vi "ENCODERS AUTO SUBVI.vi"   [LabVIEW 2011]
uses:
  Robot Global Data.vi
types:
  T1 = typedef "WPI_RobotDriveDevRef.ctl" = cluster{"DevStatus":errorcluster, "Motors[]":T2[], "Square Inputs":bool, "Max Output":dbl, "Isochronous":bool}
  T2 = typedef "WPI_MotorControlDeviceRef.ctl" = cluster{"DeviceStatus":errorcluster, "Type":enum16{"PWM", "CAN"}, "PWM":cluster{"Digital Module":T3, "PWM Channel":T4, "DeadBand":T5}, "CAN":cluster{"Device Number":u8, "Control Mode":T6, "Semaphore":T7, "Max Vout":dbl}, "Invert":bool, "TransformRef":T8, "InvTransformRef":T8}
  T3 = typedef "FPGA_TypedefDigitalModule.ctl" = enum16{"Digital Module 1", "Digital Module 2"}
  T4 = typedef "FPGA_DIOPWMChannel.ctl" = enum8{"PWM 1", "PWM 2", "PWM 3", "PWM 4", "PWM 5", "PWM 6", "PWM 7", "PWM 8", "PWM 9", "PWM 10", "Invalid"}
  T5 = typedef "WPI_PWMDeadband.ctl" = cluster{"Name":string, "maxPositivePwm":i32, "minPositivePwm":i32, "centerPwm":i32, "maxNegativePwm":i32, "minNegativePwm":i32, "angularRange":u16}
  T6 = typedef "WPI_CANJaguar_ControlMode.ctl" = enum8{"Percent VBus", "Current", "Speed", "Position", "Voltage"}
  T7 = typedef "Semaphore RefNum" = refnum<k1>
  T8 = typedef "WPI_PWMTransform_ConPane.ctl" = refnum<vi>
  T9 = typedef "WPI_DigitalInputDevRef.ctl" = cluster{"DevStatus":errorcluster, "DIO Channel":T10, "Digital Module":T3}
  T10 = typedef "FPGA_DIOChannel.ctl" = enum8{"DIO 1", "DIO 2", "DIO 3", "DIO 4", "DIO 5", "DIO 6", "DIO 7", "DIO 8", "DIO 9", "DIO 10", "DIO 11", "DIO 12", "DIO 13", "DIO 14", "Invalid"}
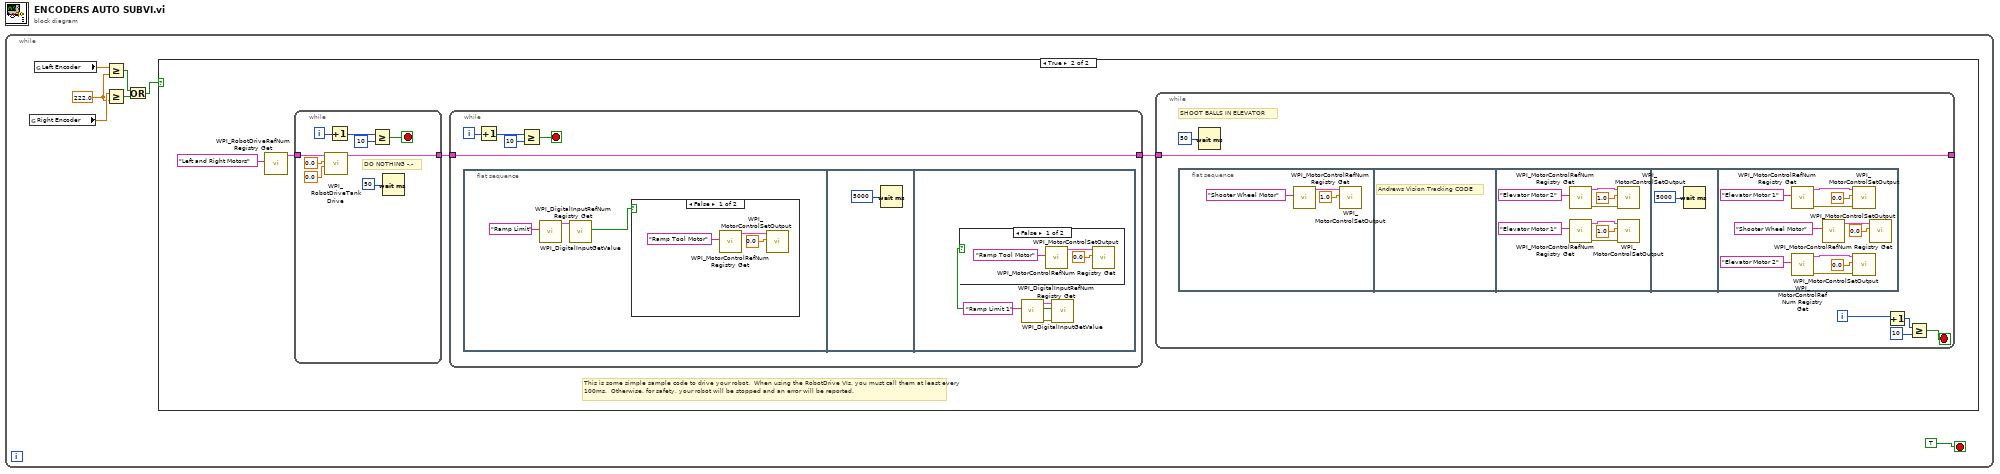
[diagram p0: block diagram]
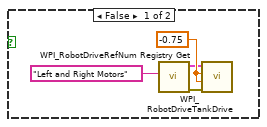
[diagram p2: hidden frame]
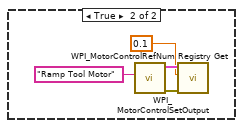
[diagram p3: hidden frame]
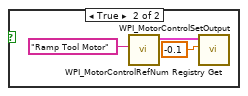
[diagram p4: hidden frame]
diagram:
  n1 = while {
    stop <- TRUE stop-if-true
    w5 = 222.0 ("y")
    n2 = global read "Robot Global Data.vi" "Right Encoder"() -> (w6:dbl)
    n3 = global read "Robot Global Data.vi" "Left Encoder"() -> (w7:dbl)
    n4 = Greater Or Equal?(x=w7, y=w5) -> (x >= y?=w4:bool)
    n5 = Greater Or Equal?(x=w6, y=w5) -> (x >= y?=w3:bool)
    n6 = Or(x=w4, y=w3) -> (x .or. y?=w2:bool)
    n7 = case shown="True" w2 {
      frame False {
        w11 = -0.75 ("Left axis value")
        n8 = call <vilib>:"WPI_RobotDriveRefNum Registry Get.vi"("refnum name"="Left and Right Motors") -> ("error out"=w9:errorcluster, "RobotDriveDevRef"=w10:T1)  [unwired: 1 in, 8 out]
        n9 = call <vilib>:"WPI_RobotDriveTankDrive.vi"("error in (no error)"=w9, "Right axis value"=w11, "Left axis value"=w11, "RobotDriveDevRef"=w10) -> ()  [unwired: 8 out]
      }
      frame True {
        # "This is some simple sample code to drive your robot.  When using the RobotDrive VIs, you must call them at least every 100ms.  Otherwise, for safety, your robot will be stopped and an error will be reported."
        n10 = call <vilib>:"WPI_RobotDriveRefNum Registry Get.vi"("refnum name"="Left and Right Motors") -> ("RobotDriveDevRef"=w14:T1)  [unwired: 1 in, 9 out]
        n11 = while {
          tunnel: w14 -> [w72]
          tunnel: [w71] -> w15
          i -> [w78]
          stop <- w76 stop-if-true
          # "DO NOTHING -.-"
          n12 = call <vilib>:"WPI_RobotDriveTankDrive.vi"("Right axis value"=0.0 ("X axis value"), "Left axis value"=0.0 ("X axis value"), "RobotDriveDevRef"=w72) -> ("RobotDriveDevRef"=w71:T1)  [unwired: 7 in, 1 out]
          n13 = Increment(x=w78) -> (x+1=w75:i32)
          n14 = Greater Or Equal?(x=w75, y=10) -> (x >= y?=w76:bool)
          n15 = Wait (ms)(milliseconds to wait=u32 50) -> ()  [unwired: 1 out]
        }
        n16 = while {
          tunnel: w15 -> [w45]
          tunnel: [w45] -> w12
          i -> [w49]
          stop <- w47 stop-if-true
          n17 = flat-sequence {
            frame #0 {
              n18 = call <vilib>:"WPI_DigitalInputRefNum Registry Get.vi"("refnum name"="Ramp Limit") -> ("DigitalInputDevRef"=w50:T9)  [unwired: 9 in, 1 out]
              n19 = call <vilib>:"WPI_DigitalInputGetValue.vi"("DigitalInputDevRef"=w50) -> ("Value"=w52:bool)  [unwired: 8 in, 2 out]
              n20 = case shown="False" w52 {
                frame False {
                  n21 = call <vilib>:"WPI_MotorControlRefNum Registry Get.vi"("refnum name"="Ramp Tool Motor") -> ("MotorControlDevRef"=w55:T2)  [unwired: 9 in, 1 out]
                  n22 = call <vilib>:"WPI_MotorControlSetOutput.vi"("Output"=0.0, "MotorControlDevRef"=w55) -> ()  [unwired: 8 in, 2 out]
                }
                frame True {
                  n23 = call <vilib>:"WPI_MotorControlRefNum Registry Get.vi"("refnum name"="Ramp Tool Motor") -> ("error out"=w58:errorcluster, "MotorControlDevRef"=w59:T2)  [unwired: 9 in]
                  n24 = call <vilib>:"WPI_MotorControlSetOutput.vi"("error in (no error)"=w58, "Output"=0.1, "MotorControlDevRef"=w59) -> ()  [unwired: 7 in, 2 out]
                }
              }
            }
            frame #1 {
              n25 = Wait (ms)(milliseconds to wait=u32 5000) -> ()  [unwired: 1 out]
            }
            frame #2 {
              n26 = call <vilib>:"WPI_DigitalInputRefNum Registry Get.vi"("refnum name"="Ramp Limit 1") -> ("error out"=w64:errorcluster, "DigitalInputDevRef"=w63:T9)  [unwired: 9 in]
              n27 = call <vilib>:"WPI_DigitalInputGetValue.vi"("error in (no error)"=w64, "DigitalInputDevRef"=w63) -> ("Value"=w61:bool)  [unwired: 7 in, 2 out]
              n28 = case shown="False" w61 {
                frame False {
                  n29 = call <vilib>:"WPI_MotorControlRefNum Registry Get.vi"("refnum name"="Ramp Tool Motor") -> ("MotorControlDevRef"=w67:T2)  [unwired: 9 in, 1 out]
                  n30 = call <vilib>:"WPI_MotorControlSetOutput.vi"("Output"=0.0, "MotorControlDevRef"=w67) -> ()  [unwired: 8 in, 2 out]
                }
                frame True {
                  n31 = call <vilib>:"WPI_MotorControlRefNum Registry Get.vi"("refnum name"="Ramp Tool Motor") -> ("MotorControlDevRef"=w68:T2)  [unwired: 9 in, 1 out]
                  n32 = call <vilib>:"WPI_MotorControlSetOutput.vi"("Output"=-0.1, "MotorControlDevRef"=w68) -> ()  [unwired: 8 in, 2 out]
                }
              }
            }
          }
          n33 = Increment(x=w49) -> (x+1=w46:i32)
          n34 = Greater Or Equal?(x=w46, y=10) -> (x >= y?=w47:bool)
        }
        n35 = while {
          tunnel: [w18] -> _
          tunnel: w12 -> [w18]
          i -> [w17]
          stop <- w16 stop-if-true
          # "SHOOT BALLS IN ELEVATOR"
          n36 = flat-sequence {
            frame #0 {
              n37 = call <vilib>:"WPI_MotorControlRefNum Registry Get.vi"("refnum name"="Shooter Wheel Motor") -> ("MotorControlDevRef"=w24:T2)  [unwired: 9 in, 1 out]
              n38 = call <vilib>:"WPI_MotorControlSetOutput.vi"("Output"=1.0, "MotorControlDevRef"=w24) -> ()  [unwired: 8 in, 2 out]
            }
            frame #1 {
              # "Andrews Vision Tracking CODE"
            }
            frame #2 {
              n39 = call <vilib>:"WPI_MotorControlRefNum Registry Get.vi"("refnum name"="Elevator Motor 2") -> ("error out"=w32:errorcluster, "MotorControlDevRef"=w31:T2)  [unwired: 9 in]
              n40 = call <vilib>:"WPI_MotorControlRefNum Registry Get.vi"("refnum name"="Elevator Motor 1") -> ("error out"=w28:errorcluster, "MotorControlDevRef"=w27:T2)  [unwired: 9 in]
              n41 = call <vilib>:"WPI_MotorControlSetOutput.vi"("error in (no error)"=w32, "Output"=1.0, "MotorControlDevRef"=w31) -> ()  [unwired: 7 in, 2 out]
              n42 = call <vilib>:"WPI_MotorControlSetOutput.vi"("error in (no error)"=w28, "Output"=1.0, "MotorControlDevRef"=w27) -> ()  [unwired: 7 in, 2 out]
            }
            frame #3 {
              n43 = Wait (ms)(milliseconds to wait=5000) -> ()  [unwired: 1 out]
            }
            frame #4 {
              n44 = call <vilib>:"WPI_MotorControlRefNum Registry Get.vi"("refnum name"="Elevator Motor 1") -> ("error out"=w40:errorcluster, "MotorControlDevRef"=w39:T2)  [unwired: 9 in]
              n45 = call <vilib>:"WPI_MotorControlRefNum Registry Get.vi"("refnum name"="Elevator Motor 2") -> ("error out"=w44:errorcluster, "MotorControlDevRef"=w43:T2)  [unwired: 9 in]
              n46 = call <vilib>:"WPI_MotorControlRefNum Registry Get.vi"("refnum name"="Shooter Wheel Motor") -> ("MotorControlDevRef"=w36:T2)  [unwired: 9 in, 1 out]
              n47 = call <vilib>:"WPI_MotorControlSetOutput.vi"("error in (no error)"=w40, "Output"=0.0, "MotorControlDevRef"=w39) -> ()  [unwired: 7 in, 2 out]
              n48 = call <vilib>:"WPI_MotorControlSetOutput.vi"("error in (no error)"=w44, "Output"=0.0, "MotorControlDevRef"=w43) -> ()  [unwired: 7 in, 2 out]
              n49 = call <vilib>:"WPI_MotorControlSetOutput.vi"("Output"=0.0, "MotorControlDevRef"=w36) -> ()  [unwired: 8 in, 2 out]
            }
          }
          n50 = Wait (ms)(milliseconds to wait=u32 50) -> ()  [unwired: 1 out]
          n51 = Increment(x=w17) -> (x+1=w20:i32)
          n52 = Greater Or Equal?(x=w20, y=10) -> (x >= y?=w16:bool)
        }
      }
    }
  }
